vi "blowfish_internals.vi"(4 "Enc/Dec":enum16{"Encipher", "Decipher"}(ring), 5 "S 4X256":u32[][](array[numeric]) format="%.0x", 6 "P 18":u32[](array[numeric]) format="%.0x", 7 "Xr":u32=305419896 format="%.0x", 8 "Xl":u32=305419896 format="%.0x") -> (2 "Xr out":u32 format="%.0x", 3 "Xl out":u32 format="%.0x")   [LabVIEW 2020]
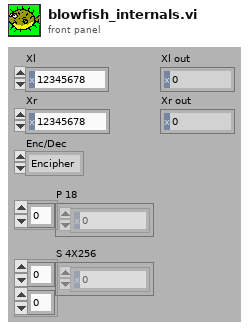
[diagram p1: front panel]
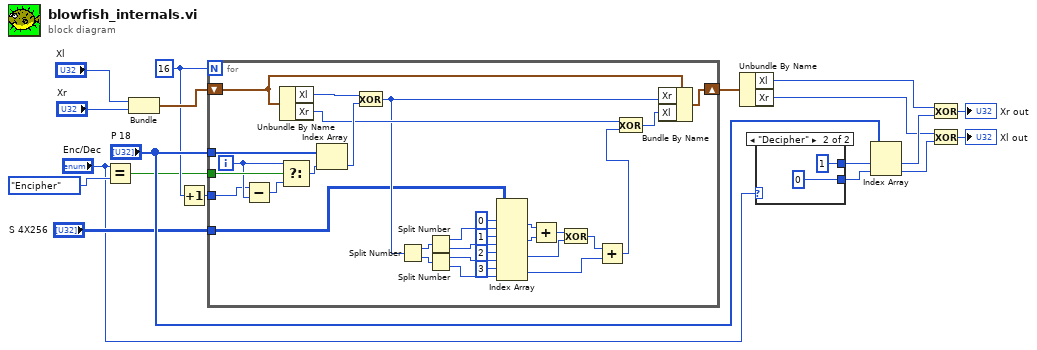
[diagram p0: block diagram]
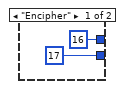
[diagram p2: hidden frame]
diagram:
  w7 = 16
  n1 = Equal?(x="Enc/Dec", y=enum16{"Encipher", "Decipher"}."Encipher") -> (x = y?=w1:bool)
  n2 = Bundle("Xl"="Xl", "Xr"="Xr") -> (w11:cluster{"Xl":u32, "Xr":u32})  [unwired: 1 in]
  n3 = Increment(x=w7) -> (x+1=w8:i32)
  n4 = for {
    N: w7 -> [_]
    shift-right: [w45] -> w14
    shift-left: w11 -> [w46]
    tunnel: "P 18" -> [w50]
    tunnel: "S 4X256" -> [w21]
    tunnel: w1 -> [w43]
    tunnel: w8 -> [w39]
    i -> [w40]
    n5 = Subtract(x=w39, y=w40) -> (x-y=w41:i32)
    n6 = Unbundle By Name(w46) -> ("Xl"=w48:u32, "Xr"=w47:u32)
    n7 = Select(t=w40, s=w43, f=w41) -> (s? t:f=w42:i32)
    n8 = Index Array(array=w50, index=w42) -> (element=w49:u32)
    n9 = Exclusive Or(1:w49, 2:w48) -> (0:w22:u32)
    n10 = Split Number(x=w22) -> (hi(x)=w38:u16, lo(x)=w37:u16)
    n11 = Split Number(x=w38) -> (hi(x)=w26:u8, lo(x)=w25:u8)
    n12 = Split Number(x=w37) -> (hi(x)=w24:u8, lo(x)=w23:u8)
    n13 = Index Array(array=w21, index (row) #1=0 ("index (row)"), index (col) #1=w26, index (row) #2=1 ("index (row)"), index (col) #2=w25, index (row) #3=2 ("index (row)"), index (col) #3=w24, index (row) #4=3 ("index (row)"), index (col) #4=w23) -> (element #1=w32:u32, element #2=w31:u32, element #3=w29:u32, element #4=w27:u32)
    n14 = Add(x=w32, y=w31) -> (x+y=w30:u32)
    n15 = Exclusive Or(1:w29, 2:w30) -> (0:w28:u32)
    n16 = Add(x=w28, y=w27) -> (x+y=w20:u32)
    n17 = Exclusive Or(1:w20, 2:w47) -> (0:w44:u32)
    n18 = Bundle By Name(cluster=w46, "Xr"=w22, "Xl"=w44) -> (w45:cluster{"Xl":u32, "Xr":u32})
  }
  n19 = Unbundle By Name(w14) -> ("Xl"=w4:u32, "Xr"=w3:u32)
  n20 = case shown="\"Decipher\"" "Enc/Dec" {
    tunnel: [17 ("f") 0 ("f")] -> w6
    tunnel: [16 ("f") 1 ("f")] -> w5
    frame "Encipher" {
    }
    frame "Decipher" {
    }
  }
  n21 = Index Array(array="P 18", index #1=w5, index #2=w6) -> (element #1=w15:u32, element #2=w17:u32)
  n22 = Exclusive Or(1:w15, 2:w4) -> (0:→"Xr out":u32)
  n23 = Exclusive Or(1:w17, 2:w3) -> (0:→"Xl out":u32)
